vi "Do.vi"(8 "error in (no error)":errorcluster, 10 "Actor in":refnum<class "Actor.lvclass">, 11 "Stop Calculation Msg":refnum<class "Stop Calculation Msg.lvclass">) -> (0 "error out":errorcluster, 2 "Actor out":refnum<class "Actor.lvclass">)   [LabVIEW 2020, in "GPU FFT Calculator.lvlib" / "Stop Calculation Msg.lvclass"]
doc: "This VI delivers the message to the actor by calling the appropriate method(s) on the actor."
uses:
  Stop Calculation Msg.lvclass
  <vilib>/ActorFramework/Actor/Actor.lvclass
  Stop Calculation Msg.lvclass/Stop Calculation Msg.ctl
  GPU FFT Calculator/GPU FFT Calculator.lvclass
  C:/Program Files/National Instruments/LabVIEW 2026/vi.lib/ActorFramework/Actor/Actor.lvclass
  53d947f1-6df8-4d9a-94e6-a85763f1ad5a.vi
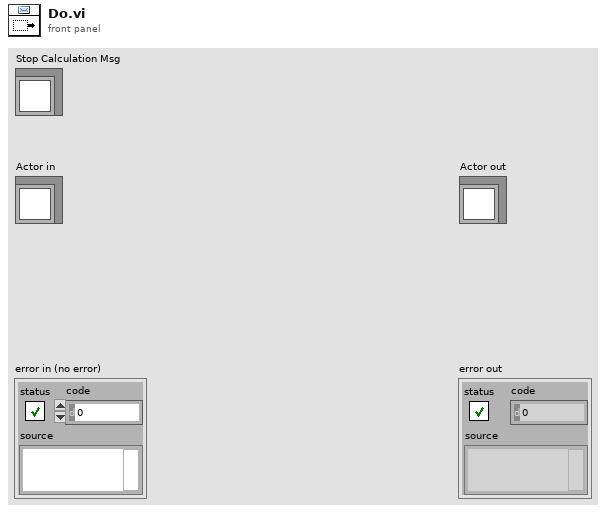
[diagram p1: front panel]
types:
  T1 = typedef "GPU FFT Calculator.lvlib/GPU FFT Calculator.lvclass/GPU Calculation Message.ctl" = cluster{"FFT Size":u64, "Batch Size":u64, "dt":dbl, "Result Buffer":refnum<data-value>, "gain":dbl, "Zoom Parameters":T2, "Upload DMA Manager":refnum<class "DMA Manager.lvclass">, "Data Buffer":refnum<data-value>, "Data Buffer GPU":refnum<class "1D Array s16.lvclass">, "GPU Metrics":T3, "df":dbl, "f0":dbl, "Zoomed Size":u64, "Result Buffer GPU":refnum<class "1D Array f32.lvclass">, "Start Time":dbl, "Batch Index":i32, "Amount of Batches":i32, "Download DMA Manager":refnum<class "DMA Manager.lvclass">}
  T2 = typedef "Simple UI.lvlib/Simple UI.lvclass/chart zoom.ctl" = cluster{"Override":bool, "f0: ":dbl, "fwidth: ":dbl}
  T3 = typedef "GPU FFT Calculator.lvlib/GPU FFT Calculator.lvclass/GPU Metrics.ctl" = cluster{"Upload Time":dbl, "Algorithm Processing Time":dbl, "Single Trace Size":u64}
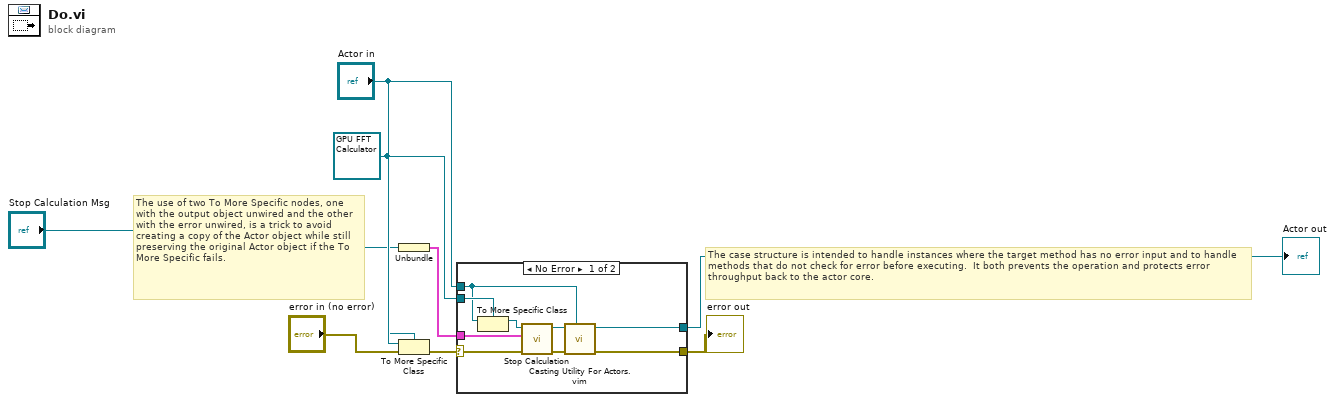
[diagram p0: block diagram]
diagram:
  w3 = refnum<class "GPU FFT Calculator.lvclass"> refnum ("Actor in")
  # "The use of two To More Specific nodes, one with the output object unwired and the other with the error unwired, is a trick to avoid creating a copy of the Actor object while still preserving the original Actor object if the To More Specific fails."
  # "The case structure is intended to handle instances where the target method has no error input and to handle methods that do not check for error before executing.  It both prevents the operation and protects error throughput back to the actor core."
  n1 = Unbundle("Stop Calculation Msg") -> (w1:T1[])
  n2 = To More Specific Class(target class=w3, reference="Actor in", error in="error in (no error)") -> (error out=w2:errorcluster)  [unwired: 1 out]
  n3 = case shown="No Error" w2 {
    selector: w2 -> [w17 w19]
    tunnel: [w11 w19] -> w8
    tunnel: [w12 w18] -> w7
    tunnel: "Actor in" -> [w14 w18]
    tunnel: w3 -> [w15 _]
    tunnel: w1 -> [w9 _]
    frame No Error {
      n4 = To More Specific Class(target class=w15, reference=w14) -> (specific class reference=w16:refnum<class "GPU FFT Calculator.lvclass">)  [unwired: 1 in, 1 out]
      n5 = call-dynamic "Stop Calculation.vi"("error in (no error)"=w17, "appended array"=w9, "GPU FFT Calculator in"=w16) -> ("error out"=w10:errorcluster, "GPU FFT Calculator out"=w13:refnum<class "GPU FFT Calculator.lvclass">)  [unwired: 7 in]
      n6 = call "Casting Utility For Actors.vim"("type"=w14, "error in (no error)"=w10, "Actor in"=w13) -> ("error out"=w11:errorcluster, "Actor out"=w12:refnum<class "Actor.lvclass">)  [unwired: 7 in]
    }
    frame Error {
      # "If type check fails, pass the original object out again."
    }
  }
  "error out" <- w8
  "Actor out" <- w7
